vi "SC10_close_shutter2.vi"(7 "error in (no error)":errorcluster, 9 "time (ms)":i32, 10 "VISA resource name":refnum<visa-resource-name>) -> (0 "error out":errorcluster, 3 "VISA resource name out":refnum<visa-resource-name>)   [LabVIEW 2010]
panel:
  out "substring":string
  out "read buffer":string
  out "return count 3":u32
  out "return count":u32
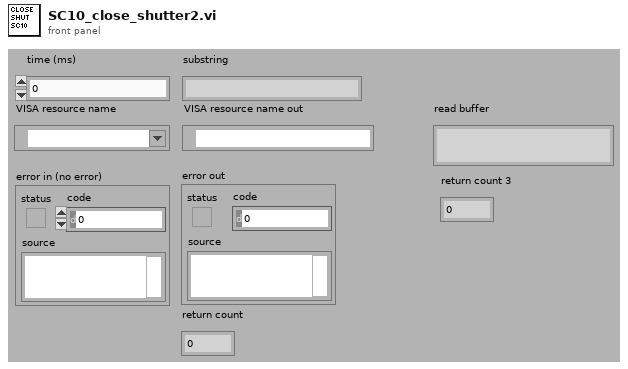
[diagram p1: front panel]
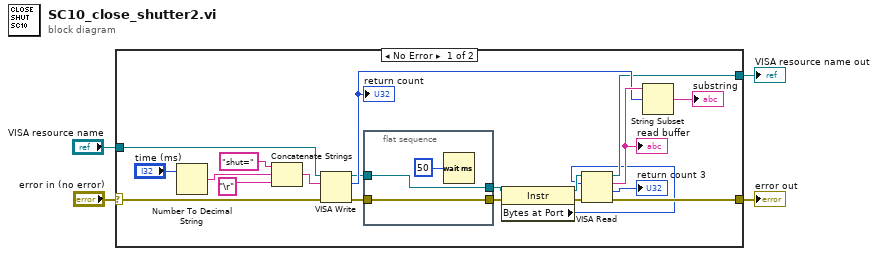
[diagram p0: block diagram]
diagram:
  n1 = case shown="No Error" "error in (no error)" {
    selector: "error in (no error)" -> [w24 w28]
    tunnel: [w11 w28] -> w3
    tunnel: [w10 w29] -> w2
    tunnel: "VISA resource name" -> [w23 w29]
    frame No Error {
      n2 = Number To Decimal String(number="time (ms)") -> (decimal integer string=w19:string)  [unwired: 1 in]
      n3 = Concatenate Strings("shut=" ("string"), w19, "\r" ("write buffer")) -> (w20:string)
      n4 = VISA Write(VISA resource name=w23, write buffer=w20, error in (no error)=w24) -> (VISA resource name out=w13:refnum<visa-resource-name>, return count=w14:u32, error out=w12:errorcluster)
      "return count" <- w14
      n5 = flat-sequence {
        tunnel: w13 -> [w26]
        tunnel: [w26] -> w7
        tunnel: w12 -> [w25]
        tunnel: [w25] -> w8
        frame #0 {
          n6 = Wait (ms)(milliseconds to wait=u32 50) -> ()  [unwired: 1 out]
        }
      }
      n7 = property class="Instr"(reference=w7, error in=w8) -> (reference out=w6:refnum<visa-resource-name>, error out=w9:errorcluster, "Bytes at Port"=w5:u32)
      n8 = VISA Read(VISA resource name=w6, byte count=w5, error in (no error)=w9) -> (VISA resource name out=w10:refnum<visa-resource-name>, read buffer=w16:string, return count=→"return count 3":u32, error out=w11:errorcluster)
      "read buffer" <- w16
      n9 = String Subset(string=w16, offset (0)=w14) -> (substring=→"substring":string)  [unwired: 1 in]
    }
    frame Error {
    }
  }
  "error out" <- w3
  "VISA resource name out" <- w2
